vi "Prog13.vi"() -> ()   [LabVIEW 2021]
panel:
  out "String 4":string
  out "String 3":string
  out "String 2":string
  out "String":string
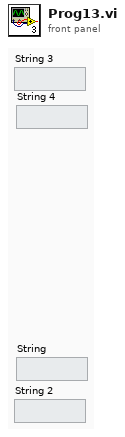
[diagram p1: front panel]
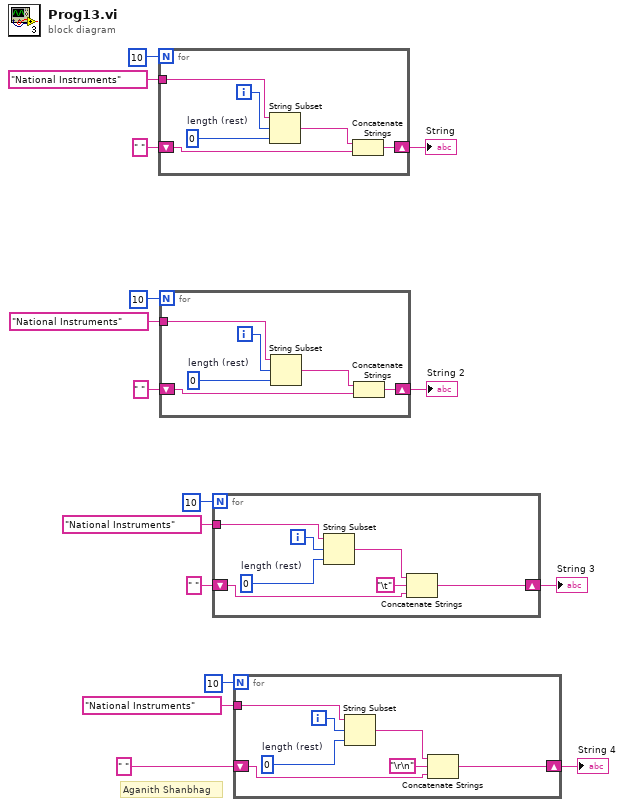
[diagram p0: block diagram]
diagram:
  # "Aganith Shanbhag"
  n1 = for {
    N: 10 -> [_]
    tunnel: "National Instruments" -> [w22]
    shift-right: [w17] -> w13
    shift-left: " " -> [w18]
    i -> [w21]
    w20 = 0  # length (rest)
    n2 = String Subset(string=w22, offset (0)=w21, length (rest)=w20) -> (substring=w19:string)
    n3 = Concatenate Strings(w19, w18) -> (w17:string)
  }
  "String" <- w13
  n4 = for {
    N: 10 -> [_]
    tunnel: "National Instruments" -> [w28]
    shift-right: [w23] -> w9
    shift-left: " " -> [w24]
    i -> [w27]
    w26 = 0  # length (rest)
    n5 = String Subset(string=w28, offset (0)=w27, length (rest)=w26) -> (substring=w25:string)
    n6 = Concatenate Strings(w25, w24) -> (w23:string)
  }
  "String 2" <- w9
  n7 = for {
    N: 10 -> [_]
    tunnel: "National Instruments" -> [w35]
    shift-right: [w31] -> w5
    shift-left: " " -> [w30]
    i -> [w34]
    w33 = 0  # length (rest)
    n8 = String Subset(string=w35, offset (0)=w34, length (rest)=w33) -> (substring=w32:string)
    n9 = Concatenate Strings "Concatenate Strings"(w32, "\t", w30) -> (w31:string)
  }
  "String 3" <- w5
  n10 = for {
    N: 10 -> [_]
    tunnel: "National Instruments" -> [w42]
    shift-right: [w38] -> w1
    shift-left: " " -> [w37]
    i -> [w41]
    w40 = 0  # length (rest)
    n11 = String Subset(string=w42, offset (0)=w41, length (rest)=w40) -> (substring=w39:string)
    n12 = Concatenate Strings "Concatenate Strings"(w39, "\r\n", w37) -> (w38:string)
  }
  "String 4" <- w1
